vi "9230_CHx3.vi"() -> ()   [LabVIEW 2018]
uses:
  <vilib>/Utility/sysdir.llb/System Directory Type.ctl
  <vilib>/DAQmx/read.llb/DAQmx Read (Analog 1D Wfm NChan NSamp).vi
  <vilib>/DAQmx/miscellaneous.llb/DAQmx Fill In Error Info.vi
  <vilib>/express/express analysis/Spectral/Block/exnSpectralBlock spectral measurements RMS poly.vi
  <vilib>/express/express analysis/Spectral/Block/exnSpectralBlock spectral measurements RMS DDT.vi
  <vilib>/ErrorRing/Error Ring.xnode
  <vilib>/express/express analysis/Spectral/XNode/ExpressSpectralMeasurementsBlockNode.xnode
  <vilib>/Utility/config.llb/NI_LVConfig.lvlib
  <vilib>/express/express signal manip/GetorSetDDTAttributes/Set DDT Attributes/Set DDT Properties.xnode
  <vilib>/express/express shared/transition.llb/Dynamic To Waveform Array.vi
  <vilib>/express/express signal manip/GetorSetDDTAttributes/Set DDT Attributes/SetT0.vi
  <vilib>/express/express shared/transition.llb/Waveform Array To Dynamic.vi
  <vilib>/express/express signal manip/GetorSetDDTAttributes/Shared VIs/XDimension.ctl
  <vilib>/express/express signal manip/GetorSetDDTAttributes/Shared VIs/GetSetShared.lvlib
  <vilib>/express/express signal manip/GetorSetDDTAttributes/Shared VIs/XDimension Enum to String.vi
  <vilib>/express/express signal manip/GetorSetDDTAttributes/Set DDT Attributes/sub Set StartTimeStamp.vi
  <vilib>/express/express signal manip/GetorSetDDTAttributes/Set DDT Attributes/Set DDT Attributes.lvlib
panel:
  out "SVING":bool caption="存檔"
  in  "Open Folder":bool
  in  "Enable Saving":bool
  out "Time":timestamp format="%<%Y/%m/%d   %H:%M:%S>T"
  in  "Tab Control":enum32{"訊號顯示", "參數設定"}(tab)
  out "CH3-Z-FFT":dynamicdata(graph)
  out "CH2-Y-FFT":dynamicdata(graph)
  out "CH1-X-FFT":dynamicdata(graph)
  out "CH3-Z-Timedomain":dynamicdata(graph)
  out "CH2-Y-Timedomain":dynamicdata(graph)
  out "CH1-X-Timedomain":dynamicdata(graph)
  out "ERROR":bool
  in  "Filter":enum16{"Bypass", "High-Pass", "Low-Pass"}(ring)
  out "DAQ Data 2":dynamicdata(graph)
  in  "Cut-Off Value":dbl=10.0
  in  "Z-Axis Sensitivity [mV/g]":dbl=14.0350854918367 format="%#.14g"
  in  "Y-Axis Sensitivity [mV/g]":dbl=13.8991380183673 format="%#.14g"
  in  "X-Axis Sensitivity [mV/g]":dbl=14.0320637122449 format="%#.14g"
  in  "DAQ Device":tag="cDAQ1Mod1"
  in  "ABORT":bool
  in  "Run":bool
  out "DAQ Stoped":bool
  out "DAQ Data":dynamicdata(graph)
  in  "PAUSE":bool
  out "DAQ Error":errorcluster
  out "DAQ (N)":i32
  out "Main (N)":i32
  out "Buffer in Queue":i32(slide) scale=0.0..100.0
  in  "Rate":dbl=12800.0 format="%#_13g"
  in  "Samples to Read":i32=6400
  # "擷取卡設定"
  # "感測器靈敏度設定"
  # "(系統開啟後修改無效)"
  # "M104009  Output Volt is 10mV/g"
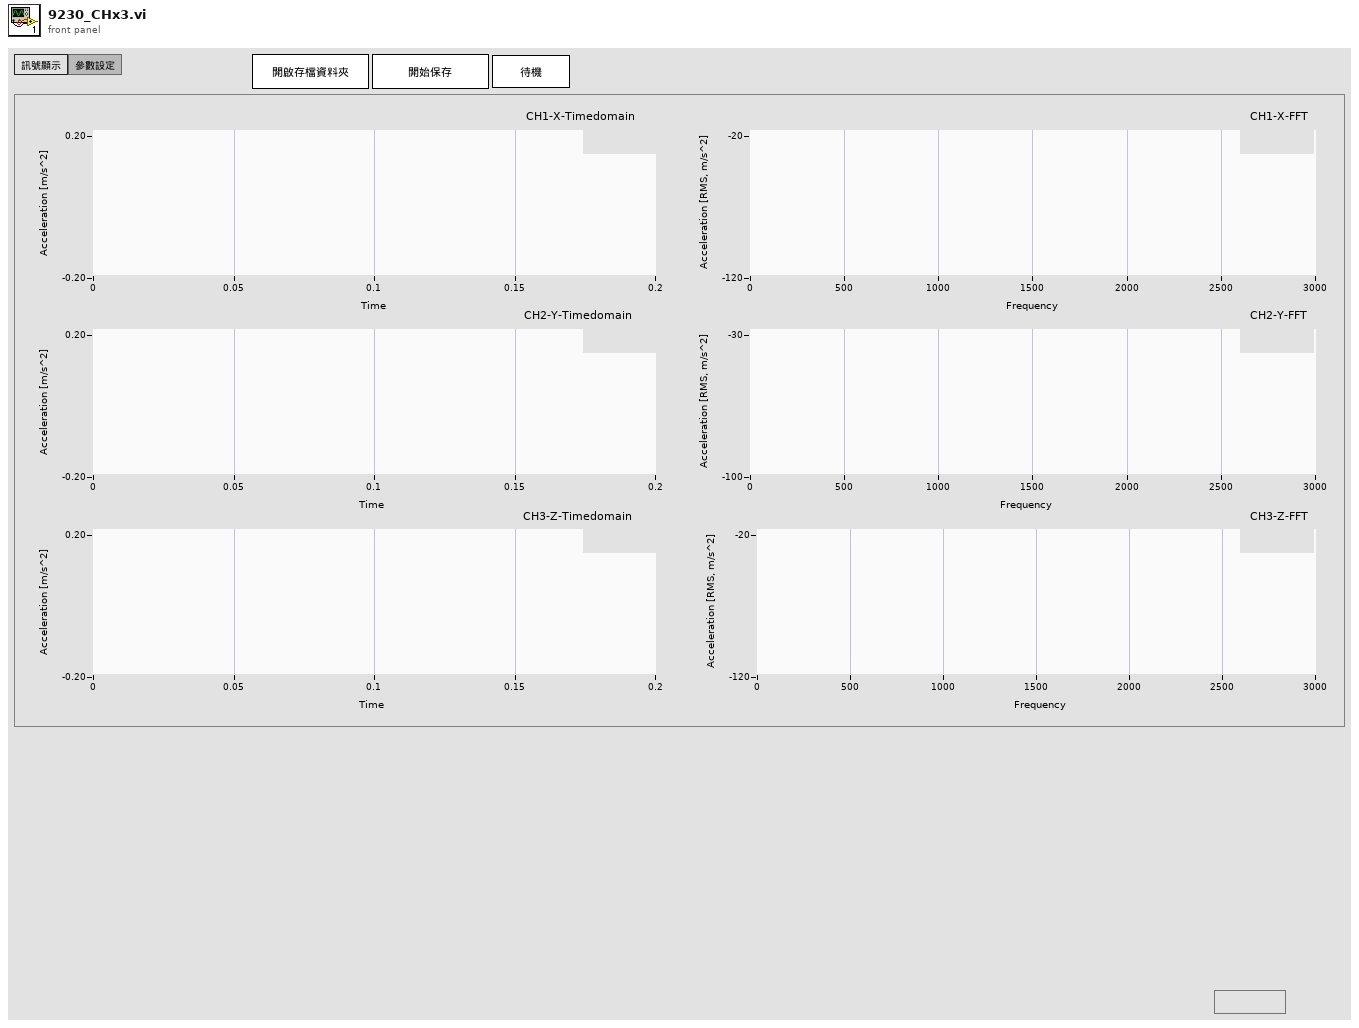
[diagram p1: front panel]
types:
  T1 = typedef "NI_LVConfig.lvlib/Config Data RefNum.ctl" = refnum<k1>
  T2 = enum8{"Enabled", "Disabled", "Disabled and Grayed Out"}
  T3 = cluster{"averaging mode":u16, "weighting mode":u16, "number of averages":u32}
  T4 = cluster{"dB On (F)":bool, "unwrap phase (F)":bool, "convert to degree (F)":bool}
  T5 = typedef "System Directory Type.ctl" = i32
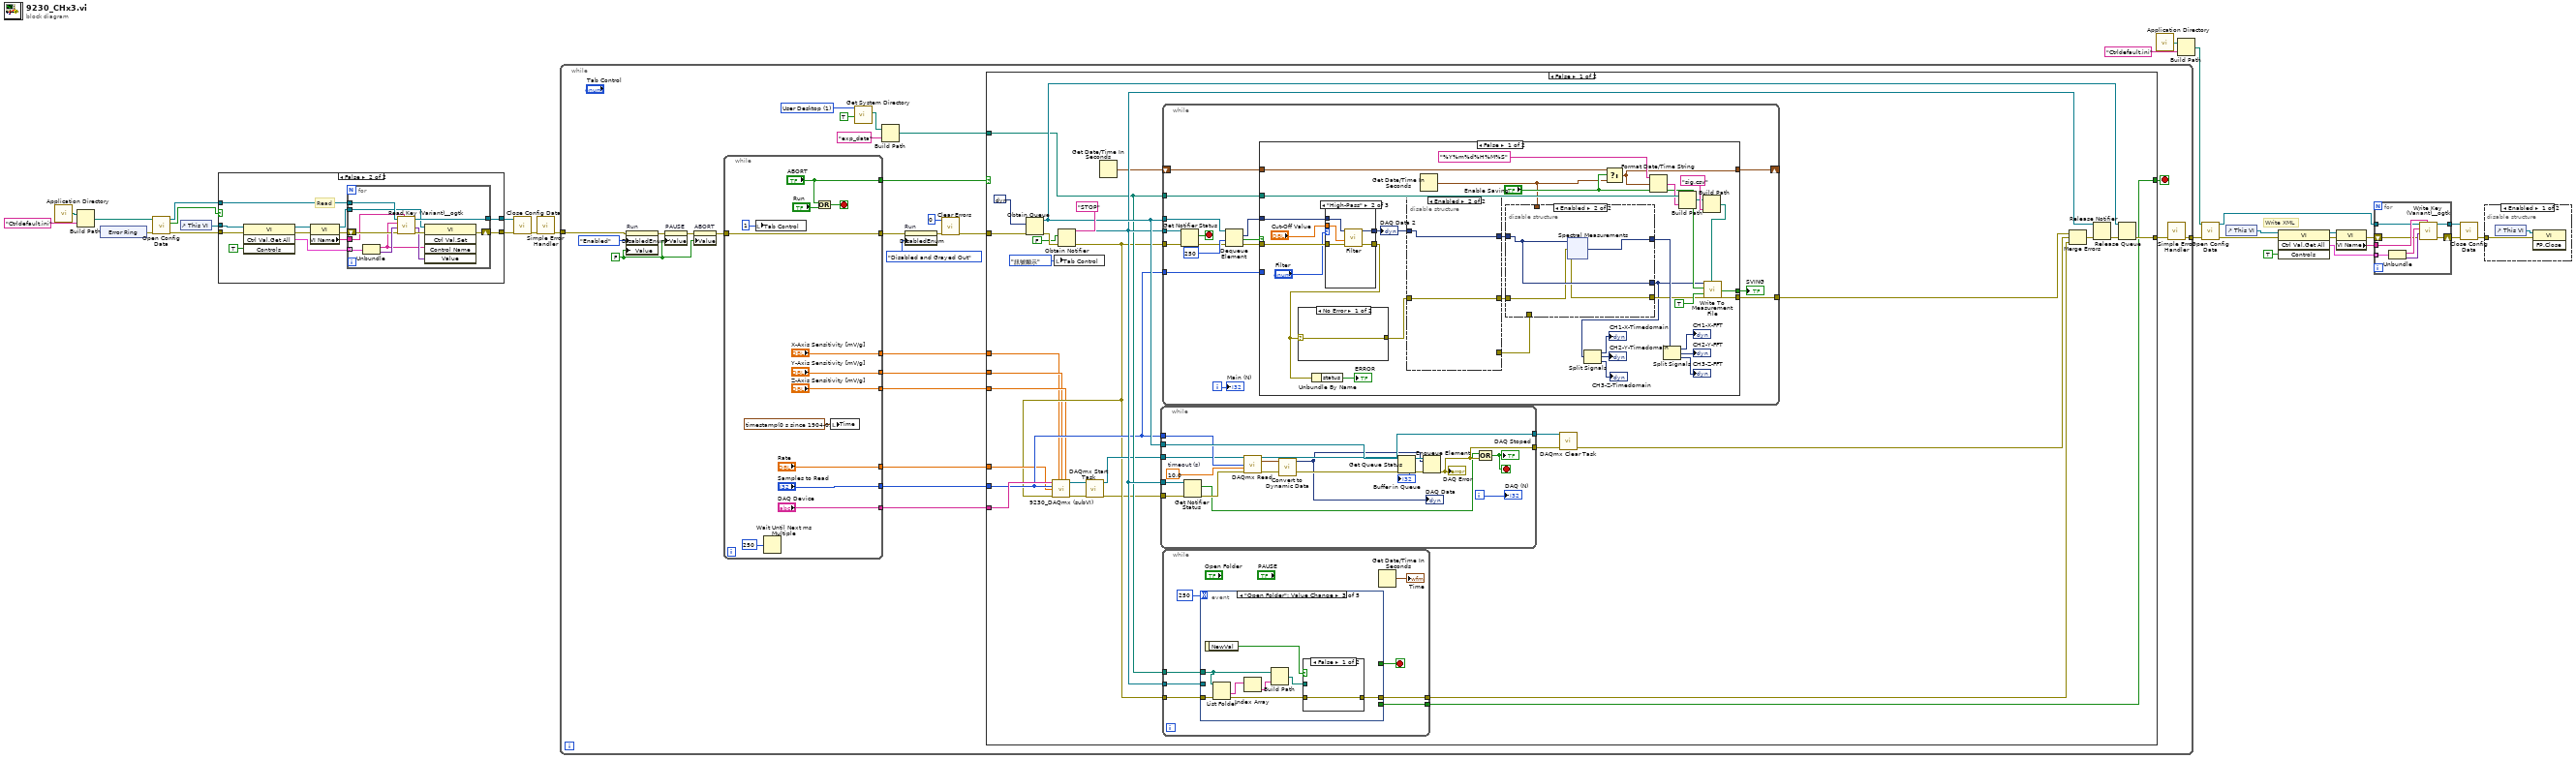
[diagram p0: block diagram]
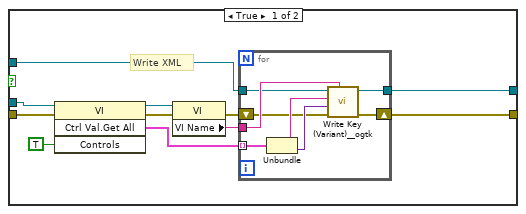
[diagram p2: hidden frame]
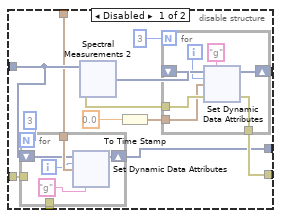
[diagram p4: hidden frame]
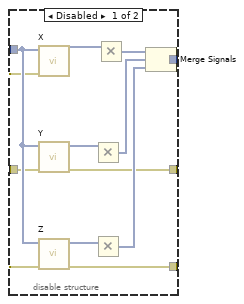
[diagram p5: hidden frame]
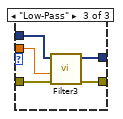
[diagram p8: hidden frame]
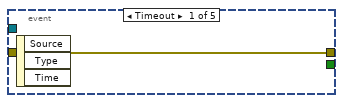
[diagram p10: hidden frame]
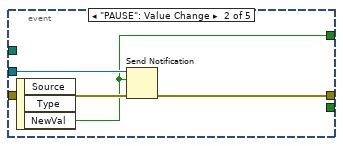
[diagram p11: hidden frame]
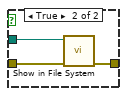
[diagram p12: hidden frame]
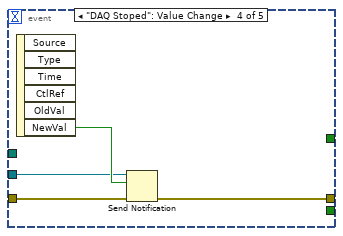
[diagram p13: hidden frame]
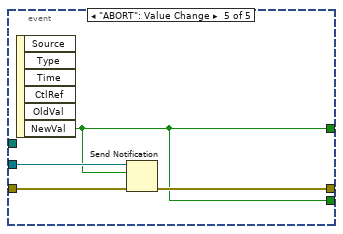
[diagram p14: hidden frame]
diagram:
  # "Write XML"
  n1 = call <vilib>:"Application Directory.vi"() -> ("Application Directory"=w1:path)
  n2 = Build Path(base path=w1, name or relative path="Ctrldefault.ini") -> (appended path=w28:path)
  n3 = xnode "Error Ring"() -> ("error out"=w20:errorcluster)
  n4 = call <vilib>:"Open Config Data.vi"("error in (no error)"=w20, "configuration file path"=w28) -> ("error out"=w25:errorcluster, "file created?"=w21:bool, "refnum"=w18:T1)  [unwired: 7 in]
  n5 = control-ref of="This VI"() -> (w19:refnum<vi>)
  n6 = case shown="False" w21 {
    tunnel: [w33 w53] -> w26
    tunnel: w25 -> [w31 w51]
    tunnel: [w29 w49] -> w24
    tunnel: w19 -> [w32 w52]
    tunnel: w18 -> [w34 w54]
    frame True {
      # "Write XML"
      n7 = invoke class="VI" method="Ctrl Val.Get All"(reference=w32, error in=w31, "Controls"=TRUE) -> (reference out=w38:refnum<vi>, error out=w37:errorcluster, "Get All Control Values Variant"=w39:cluster{"Name":string, "Variant Data":variant}[])  [unwired: 1 in, 1 out]
      n8 = property class="VI"(reference=w38, error in=w37) -> (error out=w30:errorcluster, "VI Name"=w36:string)  [unwired: 1 out]
      n9 = for {
        tunnel: w39 -> [w47] mode=indexing
        tunnel: w36 -> [w46]
        tunnel: w34 -> [w44]
        shift-right: [w43] -> w33
        shift-left: w30 -> [w41]
        tunnel: [w40] -> w29
        n10 = Unbundle(w47) -> ("Name"=w45:string, "Variant Data"=w42:variant)
        n11 = call <userlib>:"Write Key (Variant)__ogtk.vi"("section"=w46, "error in (no error)"=w41, "key-value"=w42, "key (optional)"=w45, "refnum"=w44) -> ("error out"=w43:errorcluster, "refnum out"=w40:T1)  [unwired: 5 in]
      }
    }
    frame False {
      # "Read"
      n12 = invoke class="VI" method="Ctrl Val.Get All"(reference=w52, error in=w51, "Controls"=TRUE) -> (reference out=w58:refnum<vi>, error out=w57:errorcluster, "Get All Control Values Variant"=w59:cluster{"Name":string, "Variant Data":variant}[])  [unwired: 1 in, 1 out]
      n13 = property class="VI"(reference=w58, error in=w57) -> (reference out=w48:refnum<vi>, error out=w50:errorcluster, "VI Name"=w56:string)
      n14 = for {
        tunnel: w59 -> [w70] mode=indexing
        tunnel: w56 -> [w63]
        tunnel: w54 -> [w69]
        shift-right: [w64] -> w53
        shift-left: w50 -> [w67]
        tunnel: [w66] -> w49
        tunnel: w48 -> [w62]
        n15 = Unbundle(w70) -> ("Name"=w60:string, "Variant Data"=w68:variant)
        n16 = call <userlib>:"Read Key (Variant)__ogtk.vi"("section"=w63, "error in (no error)"=w67, "type"=w68, "key (optional)"=w60, "refnum"=w69) -> ("error out"=w65:errorcluster, "key-value"=w61:variant, "refnum out"=w66:T1)  [unwired: 3 in, 1 out]
        n17 = invoke class="VI" method="Ctrl Val.Set"(reference=w62, error in=w65, "Control Name"=w60, "Value"=w61) -> (error out=w64:errorcluster)  [unwired: 1 in, 4 out]
      }
    }
  }
  n18 = call <vilib>:"Close Config Data.vi"("error in (no error)"=w26, "refnum"=w24) -> ("error out"=w23:errorcluster)  [unwired: 8 in, 1 out]
  n19 = call <vilib>:"Simple Error Handler.vi"("error in (no error)"=w23) -> ("error out"=w22:errorcluster)  [unwired: 4 in, 4 out]
  n20 = while {
    tunnel: [w96] -> w4
    tunnel: w22 -> [w76]
    stop <- w78 stop-if-true
    w86 = T5 1 items=["User Home"=0, "User Desktop"=1, "User Documents"=2, "User Application Data"=3, "User Preferences"=4, "User Temporary"=5, "Public Documents"=6, "Public Application Data"=7, "Public Preferences"=8, "Public Cache"=13, "System Core Libraries"=9, "System Installed Libraries"=10, "Application Files"=11, "Boot Volume Root"=12] ("system directory type")
    w90 = FALSE ("stop 3")
    n21 = property on="Run" class="Bool (strict)"(error in=w76, "DisabledEnum"=T2."Enabled" ("Disabled"), "Value"=w90) -> (error out=w93:errorcluster)  [unwired: 1 in, 1 out]
    n22 = property on="PAUSE" class="Bool (strict)"(error in=w93, "Value"=w90) -> (error out=w92:errorcluster)  [unwired: 1 in, 1 out]
    n23 = property on="ABORT" class="Bool (strict)"(error in=w92, "Value"=w90) -> (error out=w91:errorcluster)  [unwired: 1 in, 1 out]
    n24 = while {
      tunnel: [w368] -> w75
      tunnel: w91 -> [w368]
      tunnel: ["Samples to Read"] -> w77
      tunnel: ["Rate"] -> w81
      tunnel: ["DAQ Device"] -> w79
      tunnel: ["ABORT"] -> w74
      tunnel: ["Z-Axis Sensitivity [mV/g]"] -> w73
      tunnel: ["Y-Axis Sensitivity [mV/g]"] -> w72
      tunnel: ["X-Axis Sensitivity [mV/g]"] -> w71
      stop <- w361 stop-if-true
      n25 = local write "Tab Control"(1) -> ()
      n26 = Wait Until Next ms Multiple(millisecond multiple=u32 250) -> ()  [unwired: 1 out]
      n27 = Or(x="ABORT", y="Run") -> (x .or. y?=w361:bool)
      n28 = local write "Time"(timestamp(0 s since 1904-01-01) ("Time 2")) -> ()
    }
    n29 = call <vilib>:"Get System Directory.vi"("create directory if not found? (F)"=TRUE, "system directory type"=w86) -> ("system directory"=w88:path)  [unwired: 9 in]
    n30 = Build Path(base path=w88, name or relative path="exp_data") -> (appended path=w85:path)
    n31 = property on="Run" class="Bool (strict)"(error in=w75, "DisabledEnum"=T2."Disabled and Grayed Out" ("Disabled")) -> (error out=w83:errorcluster)  [unwired: 1 in, 1 out]
    n32 = call <vilib>:"Clear Errors.vi"("error in (no error)"=w83, "specific error code to clear (0: all)"=0) -> ("error out"=w82:errorcluster)  [unwired: 4 in, 1 out]
    n33 = case shown="False" w74 {
      selector: w74 -> [_ w354]
      tunnel: w82 -> [w122 w355]
      tunnel: w81 -> [w102 _]
      tunnel: [w119 w355] -> w80
      tunnel: w79 -> [w104 _]
      tunnel: [w116 w354] -> w78
      tunnel: w77 -> [w103 _]
      tunnel: w85 -> [w115 _]
      tunnel: w73 -> [w99 _]
      tunnel: w72 -> [w98 _]
      tunnel: w71 -> [w97 _]
      frame False {
        n34 = Obtain Queue(element data type=dynamicdata [] ("data"), error in (no error)=w122) -> (queue out=w121:refnum<queue>, error out=w125:errorcluster)  [unwired: 3 in, 1 out]
        n35 = local write "Tab Control"(enum32{"訊號顯示", "參數設定"}."訊號顯示" ("Tab Control")) -> ()
        n36 = Obtain Notifier(name (unnamed)="STOP", notification data type=FALSE, error in (no error)=w125) -> (notifier out=w117:refnum<notifier>, error out=w101:errorcluster)  [unwired: 1 in, 1 out]
        n37 = call "9230_DAQmx (subVI).vi"("DAQ Device"=w104, "ai0_sensitivity"=w97, "ai1_sensitivity"=w98, "ai2_sensitivity"=w99, "number of samples"=w103, "rate"=w102, "error in"=w101) -> ("task out"=w106:refnum<k21>, "error out"=w105:errorcluster)  [unwired: 7 in]
        n38 = call <vilib>:"DAQmx Start Task.vi"("task/channels in"=w106, "error in"=w105) -> ("task out"=w107:refnum<k21>, "error out"=w100:errorcluster)  [unwired: 12 in]
        n39 = Get Date/Time In Seconds() -> (seconds since 1Jan1904=w114:timestamp)
        n40 = while {
          tunnel: w121 -> [w318]
          tunnel: [w311] -> w109
          tunnel: w100 -> [w315]
          tunnel: w117 -> [w313]
          tunnel: w103 -> [w310]
          tunnel: [w308] -> w110
          tunnel: w107 -> [w307]
          i -> [w320]
          stop <- w312 stop-if-true
          w305 = 10.0  # timeout (s)
          n41 = Get Notifier Status(notifier=w313, error in (no error)=w315) -> (current notification=w303:bool, error out=w314:errorcluster)  [unwired: 3 out]
          n42 = call-poly <vilib>:"DAQmx Read.vi"("task/channels in"=w307, "number of samples per channel"=w310, "timeout"=w305, "error in"=w314) -> ("task out"=w308:refnum<k21>, "data"=w306:waveform(dbl)[], "error out"=w309:errorcluster)  [unwired: 9 in]
          n43 = call "Convert to Dynamic Data"("Array of Waveforms"=w306) -> ("Dynamic Data Type"=w304:dynamicdata)  [unwired: 3 in]
          "DAQ Data" <- w304
          n44 = Get Queue Status(queue=w318, error in (no error)=w309) -> (queue out=w317:refnum<queue>, error out=w316:errorcluster, # elements in queue=→"Buffer in Queue":i32)  [unwired: 1 in, 5 out]
          n45 = Enqueue Element(queue=w317, element=w304, error in (no error)=w316) -> (error out=w311:errorcluster)  [unwired: 1 in, 2 out]
          "DAQ Error" <- w311
          n46 = Compound Arithmetic op=OR(w303, w311) -> (w312:bool)
          "DAQ Stoped" <- w312
          "DAQ (N)" <- w320
        }
        n47 = while {
          tunnel: w121 -> [w136]
          tunnel: w101 -> [w131]
          tunnel: w117 -> [w137]
          tunnel: w103 -> [w134]
          tunnel: w115 -> [w133]
          shift-right: [w128] -> _
          shift-left: w114 -> [w129]
          tunnel: [w127] -> w112
          i -> [w142]
          stop <- w138 stop-if-true
          n48 = Get Notifier Status(notifier=w137, error in (no error)=w131) -> (current notification=w138:bool, error out=w130:errorcluster)  [unwired: 3 out]
          n49 = Dequeue Element(queue=w136, timeout in ms (-1)=250, error in (no error)=w130) -> (element=w140:dynamicdata, timed out?=w135:bool, error out=w139:errorcluster)  [unwired: 1 out]
          n50 = case shown="False" w135 {
            tunnel: w140 -> [w171 _]
            tunnel: w139 -> [w174 w302]
            tunnel: [w175 w302] -> w127
            tunnel: w134 -> [_ _]
            tunnel: w133 -> [w173 _]
            tunnel: [w172 _] -> w132
            tunnel: w129 -> [w160 w301]
            tunnel: [w156 w301] -> w128
            frame False {
              n51 = case shown="\"High-Pass\"" "Filter" {
                tunnel: w174 -> [w289 w295 w300]
                tunnel: [w290 w294 w299] -> w163
                tunnel: "Cut-Off Value" -> [_ w293 w298]
                tunnel: w171 -> [w290 w292 w297]
                tunnel: [w289 w291 w296] -> w153
                frame "Bypass", Default {
                }
                frame "High-Pass" {
                  n52 = call "Filter"("error in (no error)"=w295, "Lower Cut-Off"=w293, "Signal"=w292) -> ("error out"=w291:errorcluster, "Filtered Signal"=w294:dynamicdata)  [unwired: 7 in]
                }
                frame "Low-Pass" {
                  n53 = call "Filter3"("error in (no error)"=w300, "Lower Cut-Off"=w298, "Signal"=w297) -> ("error out"=w296:errorcluster, "Filtered Signal"=w299:dynamicdata)  [unwired: 7 in]
                }
              }
              "DAQ Data 2" <- w163
              n54 = case shown="No Error" w153 {
                selector: w153 -> [w288 _]
                tunnel: [w288 _] -> w155
                frame No Error {
                }
                frame Error {
                }
              }
              n55 = Unbundle By Name(w153) -> ("status"=→"ERROR":bool)
              n56 = disable-structure shown="Enabled" {
                disable-tunnel: w163 -> [w283 w287]
                disable-tunnel: w155 -> [w278 w286]
                disable-tunnel: [w274 w287] -> w151
                disable-tunnel: [w273 w286] -> w150
                disable-tunnel: [w272 _] -> w149
                frame Disabled {
                  n57 = call "X"("error in (no error)"=w278, "Signals"=w283) -> ("Signal Out"=w285:dynamicdata)  [unwired: 8 in, 1 out]
                  n58 = call "Y"("error in (no error)"=w278, "Signals"=w283) -> ("error out"=w273:errorcluster, "Signal Out"=w282:dynamicdata)  [unwired: 8 in]
                  n59 = call "Z"("error in (no error)"=w278, "Signals"=w283) -> ("error out"=w272:errorcluster, "Signal Out"=w280:dynamicdata)  [unwired: 8 in]
                  n60 = Multiply(x=w282) -> (y=w281:dbl, x*y=w277:dynamicdata)
                  n61 = Multiply(x=w280) -> (y=w279:dbl, x*y=w276:dynamicdata)
                  n62 = Multiply(x=w285) -> (y=w284:dbl, x*y=w275:dynamicdata)
                  n63 = Merge Signals(w275, w277, w276) -> (w274:dynamicdata)
                }
                frame Enabled {
                }
              }
              n64 = Get Date/Time In Seconds() -> (seconds since 1Jan1904=w148:timestamp)
              n65 = disable-structure shown="Enabled" {
                disable-tunnel: [w186 w261] -> w152
                disable-tunnel: w151 -> [w185 w260]
                disable-tunnel: w150 -> [w183 w259]
                disable-tunnel: w149 -> [w182 _]
                disable-tunnel: w148 -> [w181 _]
                disable-tunnel: [w177 w258] -> w147
                disable-tunnel: [w176 w260] -> w146
                frame Disabled {
                  n66 = for {
                    N: 3 -> [_]
                    tunnel: w181 -> [w193]
                    tunnel: w183 -> [_]
                    tunnel: w182 -> [_]
                    shift-right: [w189] -> w176
                    shift-left: w185 -> [w192]
                    i -> [w190]
                    n67 = xnode ("Set Dynamic Data Attributes")("Signals In"=w192, "Signal Index"=w190, "Unit"="g", "Timestamp"=w193, "Start Timestamp"=w193) -> ("Signals Out"=w189:dynamicdata)  [unwired: 2 in, 1 out]
                  }
                  n68 = xnode ("Spectral Measurements 2")("Signals"=w185) -> ("FFT - (RMS)"=w188:dynamicdata, "error out"=w180:errorcluster)  [unwired: 1 in, 1 out]
                  n69 = To Time Stamp(1:0.0) -> (0:w179:timestamp)
                  n70 = for {
                    N: 3 -> [_]
                    shift-right: [w223] -> w186
                    shift-left: w188 -> [w225]
                    tunnel: w180 -> [w222]
                    tunnel: w179 -> [w220]
                    tunnel: [w221] -> w177
                    i -> [w224]
                    n71 = xnode ("Set Dynamic Data Attributes")("Signals In"=w225, "error in"=w222, "Signal Index"=w224, "Timestamp"=w220, "Unit"="g") -> ("Signals Out"=w223:dynamicdata, "error out"=w221:errorcluster)  [unwired: 1 in]
                  }
                }
                frame Enabled {
                  n72 = xnode ("Spectral Measurements")("Signals"=w260, "error in (no error)"=w259) -> ("FFT - (RMS)"=w261:dynamicdata, "error out"=w258:errorcluster)  [unwired: 1 out]
                }
              }
              n73 = Split Signals(w146) -> (→"CH1-X-Timedomain":dynamicdata, →"CH2-Y-Timedomain":dynamicdata, →"CH3-Z-Timedomain":dynamicdata)  [unwired: 3 in]
              n74 = Select(t=w160, s="Enable Saving", f=w148) -> (s? t:f=w156:timestamp)
              n75 = Format Date/Time String(time format string (%c)="%Y%m%d%H%M%S", seconds (now)=w156) -> (date/time string=w159:string)  [unwired: 1 in]
              n76 = Split Signals(w152) -> (→"CH1-X-FFT":dynamicdata, →"CH2-Y-FFT":dynamicdata, →"CH3-Z-FFT":dynamicdata)  [unwired: 3 in]
              n77 = Build Path(base path=w173, name or relative path=w159) -> (appended path=w162:path)
              n78 = Build Path(base path=w162, name or relative path="sig.csv") -> (appended path=w164:path)
              n79 = call "Write To Measurement File"("Signals"=w146, "Enable"="Enable Saving", "new_file"=TRUE, "error in (no error)"=w147, "Filename"=w164) -> ("Saving Data"=w172:bool, "error out"=w175:errorcluster)  [unwired: 12 in, 1 out]
            }
            frame True {
            }
          }
          "SVING" <- w132
          "Main (N)" <- w142
        }
        n80 = while {
          tunnel: w101 -> [w328]
          tunnel: [w327] -> w126
          tunnel: w117 -> [w325]
          tunnel: [w322] -> w116
          tunnel: w115 -> [w321]
          stop <- w323 stop-if-true
          n81 = event shown="[2] \"Open Folder\": Value Change" {
            selector: _ -> [_ _ _ _ _]
            dyn-events: _ -> [_ _ _ _ _]
            timeout: 250 -> [_ _ _ _ _]
            tunnel: w328 -> [w329 w333 w339 w349 w353]
            tunnel: [w329 w332 w340 w346 w352] -> w327
            tunnel: w325 -> [_ w331 _ w347 w351]
            tunnel: [_ w330 _ _ w350] -> w323
            tunnel: [_ _ _ _ w350] -> w322
            tunnel: w321 -> [_ _ w334 _ _]
            event Timeout {
              n82 = event-data() -> ()  [unwired: 1 in, 3 out]
            }
            event "PAUSE": Value Change {
              n83 = event-data() -> ("NewVal"=w330:bool)  [unwired: 1 in, 2 out]
              n84 = Send Notification(notification=w330, notifier=w331, error in (no error)=w333) -> (error out=w332:errorcluster)  [unwired: 1 out]
            }
            event "Open Folder": Value Change {
              n85 = event-data() -> ("NewVal"=w341:bool)  [unwired: 1 in]
              n86 = List Folder(path=w334, error in=w339) -> (folder names=w337:string[], error out=w338:errorcluster)  [unwired: 2 in, 2 out]
              n87 = Index Array(array=w337) -> (element=w336:string)  [unwired: 1 in]
              n88 = Build Path(base path=w334, name or relative path=w336) -> (appended path=w335:path)
              n89 = case shown="False" w341 {
                tunnel: w338 -> [w342 w345]
                tunnel: w335 -> [_ w344]
                tunnel: [w342 w343] -> w340
                frame False {
                }
                frame True {
                  n90 = call <vilib>:"Show in File System.vi"("error in (no error)"=w345, "file or directory path"=w344) -> ("error out"=w343:errorcluster)  [unwired: 9 in]
                }
              }
            }
            event "DAQ Stoped": Value Change {
              n91 = event-data() -> ("NewVal"=w348:bool)  [unwired: 1 in, 5 out]
              n92 = Send Notification(notification=w348, notifier=w347, error in (no error)=w349) -> (error out=w346:errorcluster)  [unwired: 1 out]
            }
            event "ABORT": Value Change {
              n93 = event-data() -> ("NewVal"=w350:bool)  [unwired: 1 in, 5 out]
              n94 = Send Notification(notification=w350, notifier=w351, error in (no error)=w353) -> (error out=w352:errorcluster)  [unwired: 1 out]
            }
          }
          n95 = Get Date/Time In Seconds() -> (seconds since 1Jan1904=→"Time":timestamp)
        }
        n96 = call <vilib>:"DAQmx Clear Task.vi"("task in"=w110, "error in"=w109) -> ("error out"=w108:errorcluster)  [unwired: 13 in]
        n97 = Merge Errors(w112, w108, w126) -> (w118:errorcluster)
        n98 = Release Notifier(notifier=w117, error in (no error)=w118) -> (error out=w120:errorcluster)  [unwired: 1 in, 2 out]
        n99 = Release Queue(queue=w121, error in (no error)=w120) -> (error out=w119:errorcluster)  [unwired: 1 in, 2 out]
      }
      frame True {
      }
    }
    n100 = call <vilib>:"Simple Error Handler.vi"("error in (no error)"=w80) -> ("error out"=w96:errorcluster)  [unwired: 4 in, 4 out]
  }
  n101 = call <vilib>:"Application Directory.vi"() -> ("Application Directory"=w2:path)
  n102 = Build Path(base path=w2, name or relative path="Ctrldefault.ini") -> (appended path=w11:path)
  n103 = call <vilib>:"Open Config Data.vi"("error in (no error)"=w4, "configuration file path"=w11) -> ("error out"=w14:errorcluster, "refnum"=w17:T1)  [unwired: 7 in, 1 out]
  n104 = control-ref of="This VI"() -> (w16:refnum<vi>)
  n105 = invoke class="VI" method="Ctrl Val.Get All"(reference=w16, error in=w14, "Controls"=TRUE) -> (reference out=w9:refnum<vi>, error out=w8:errorcluster, "Get All Control Values Variant"=w10:cluster{"Name":string, "Variant Data":variant}[])  [unwired: 1 in, 1 out]
  n106 = property class="VI"(reference=w9, error in=w8) -> (error out=w5:errorcluster, "VI Name"=w7:string)  [unwired: 1 out]
  n107 = for {
    tunnel: w10 -> [w376] mode=indexing
    tunnel: w7 -> [w375]
    tunnel: w17 -> [w373]
    shift-right: [w372] -> w13
    shift-left: w5 -> [w370]
    tunnel: [w369] -> w15
    n108 = Unbundle(w376) -> ("Name"=w374:string, "Variant Data"=w371:variant)
    n109 = call <userlib>:"Write Key (Variant)__ogtk.vi"("section"=w375, "error in (no error)"=w370, "key-value"=w371, "key (optional)"=w374, "refnum"=w373) -> ("error out"=w372:errorcluster, "refnum out"=w369:T1)  [unwired: 5 in]
  }
  n110 = call <vilib>:"Close Config Data.vi"("error in (no error)"=w13, "refnum"=w15) -> ("error out"=w3:errorcluster)  [unwired: 8 in, 1 out]
  n111 = disable-structure shown="Enabled" {
    disable-tunnel: w3 -> [w377 _]
    frame Enabled {
      n112 = control-ref of="This VI"() -> (w378:refnum<vi>)
      n113 = invoke class="VI" method="FP.Close"(reference=w378, error in=w377) -> ()  [unwired: 1 in, 3 out]
    }
    frame Disabled {
    }
  }
